vi "Autonomous Independent.vi"() -> ()   [LabVIEW 2014]
doc: "This VI is called when autonomous begins, and will automatically be terminated when autonomous ends. You can carry out timed or sensor driven robot movement independently without needing to return to the caller."
uses:
  <vilib>/Rock Robotics/WPI/Joystick/WPI_JoystickGetSetRefNum.vi
  <vilib>/Rock Robotics/Network Tables/SD Read Boolean.vi
panel:
  in  "input cluster":T1
  # "Be sure to right-click and choose Data Operations>>Make Current Value default if you want to save the array values with the VI"
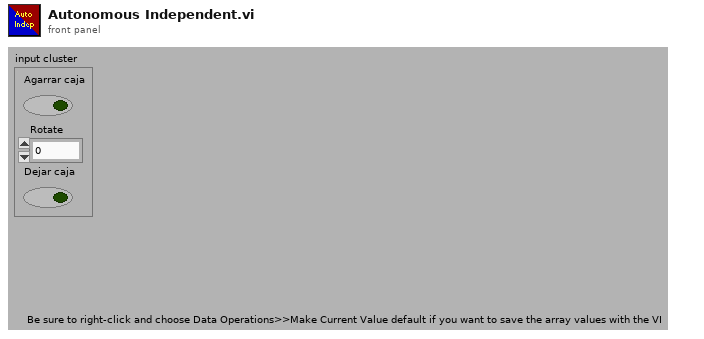
[diagram p1: front panel]
types:
  T1 = cluster{"Agarrar caja":bool, "Rotate":dbl, "Dejar caja":bool}
  T2 = enum16{"GTFO", "Drop the beat", "Moonwalk", "Stare at the box", "Kiss the Wall", "Take that motherfucker"}
  T3 = typedef "WPI_JoystickDevRef.ctl" = cluster{"Device":T4}
  T4 = typedef "WPI_JoystickDeviceEnum.ctl" = enum16{"USB 0", "USB 1", "USB 2", "USB 3", "USB 4", "USB 5"}
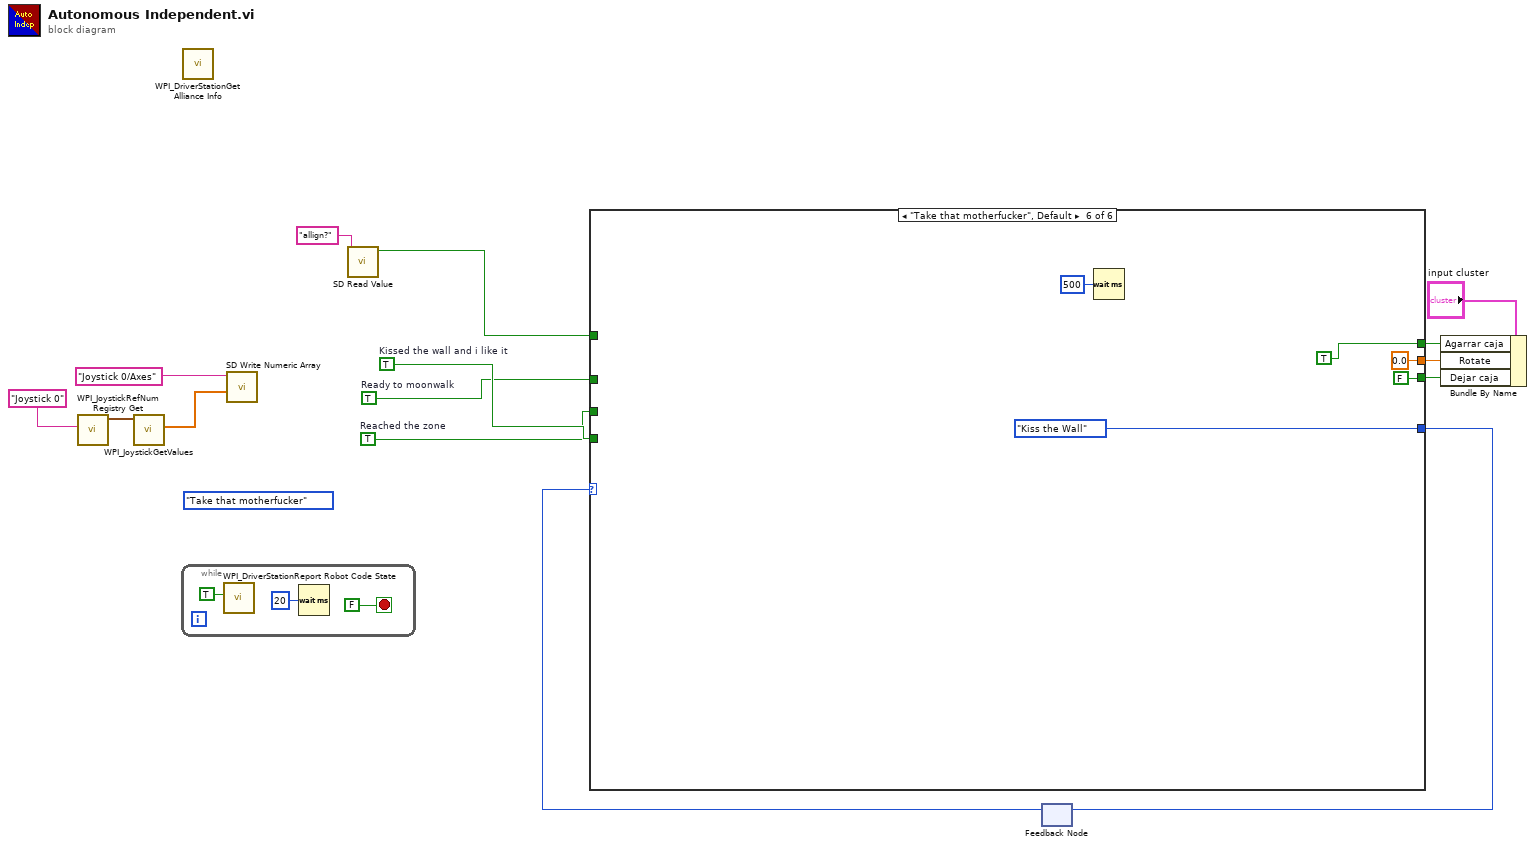
[diagram p0: block diagram]
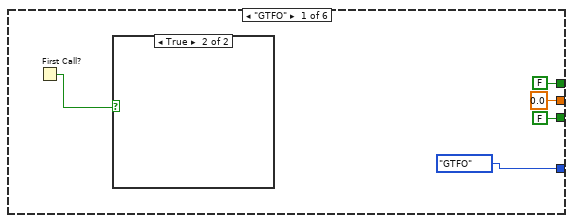
[diagram p2: hidden frame]
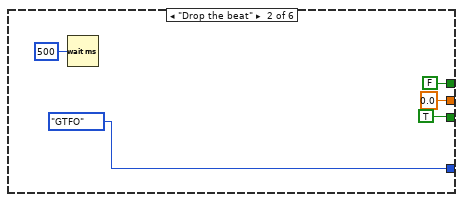
[diagram p4: hidden frame]
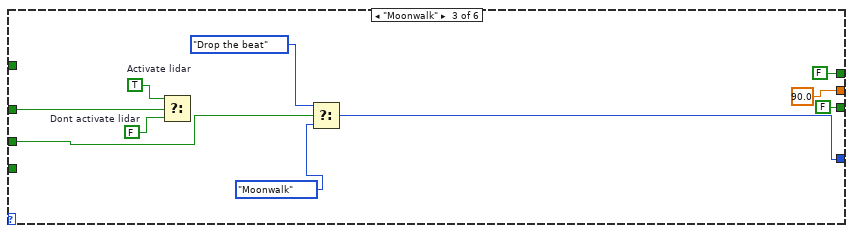
[diagram p5: hidden frame]
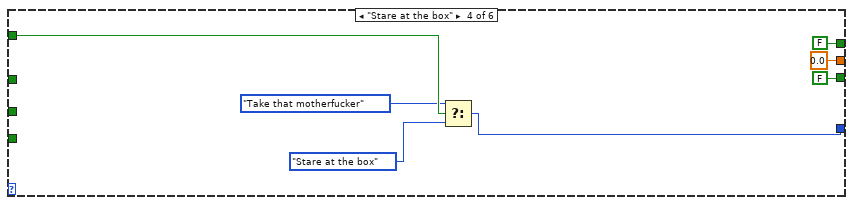
[diagram p6: hidden frame]
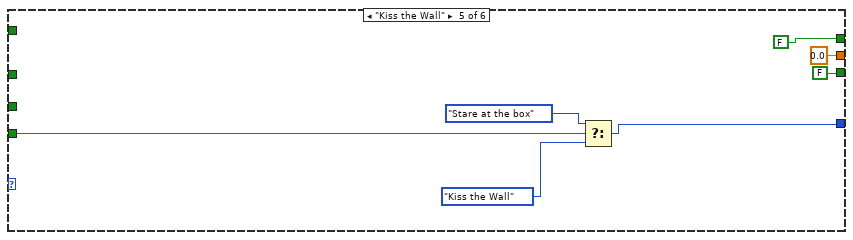
[diagram p7: hidden frame]
diagram:
  w2 = TRUE  # Reached the zone
  w3 = TRUE  # Ready to moonwalk
  w7 = TRUE  # Kissed the wall and i like it
  (unwired) T2."Take that motherfucker"
  n1 = call <vilib>:"WPI_JoystickRefNum Registry Get.vi"("refnum name"="Joystick 0") -> ("JoystickDevRef"=w14:T3)  [unwired: 1 in, 9 out]
  n2 = call <vilib>:"WPI_JoystickGetValues.vi"("JoystickDevRef"=w14) -> ("Axes"=w12:dbl[])  [unwired: 6 in, 4 out]
  n3 = while {
    stop <- FALSE stop-if-true
    n4 = call <vilib>:"WPI_DriverStationReport Robot Code State.vi"("Autonomous"=TRUE) -> ()  [unwired: 10 in, 1 out]
    n5 = Wait (ms)(milliseconds to wait=u32 20) -> ()  [unwired: 1 out]
  }
  n6 = call <vilib>:"WPI_DriverStationGet Alliance Info.vi"() -> ()  [unwired: 12 out]
  n7 = call <vilib>:"SD Write Numeric Array.vi"("Numeric Array"=w12, "Name"="Joystick 0/Axes") -> ()  [unwired: 8 in, 2 out]
  n8 = call-poly <vilib>:"SD Read Value.vi"("Name"="allign?") -> ("Boolean"=w5:bool)  [unwired: 8 in, 2 out]
  n9 = feedback #1() -> (w8:T2)  [unwired: 1 in]
  n10 = case shown="\"Take that motherfucker\", Default" w8 {
    tunnel: [FALSE FALSE FALSE FALSE FALSE TRUE] -> w10
    tunnel: [T2."GTFO" T2."GTFO" w31 w42 w50 T2."Kiss the Wall"] -> w9
    tunnel: w7 -> [_ _ _ _ w48 _]
    tunnel: w5 -> [_ _ _ w45 _ _]
    tunnel: [0.0 0.0 90.0 0.0 0.0 0.0] -> w4
    tunnel: w3 -> [_ _ w37 _ _ _]
    tunnel: w2 -> [_ _ w34 _ _ _]
    tunnel: [FALSE TRUE FALSE FALSE FALSE FALSE] -> w1
    frame "GTFO" {
      n11 = First Call?() -> (First Call?: T/F=w19:bool)
      n12 = case shown="True" w19 {
        frame False {
        }
        frame True {
        }
      }
    }
    frame "Drop the beat" {
      n13 = Wait (ms)(milliseconds to wait=u32 500) -> ()  [unwired: 1 out]
    }
    frame "Moonwalk" {
      w35 = TRUE  # Activate lidar
      w36 = FALSE  # Dont activate lidar
      n14 = Select(t=w35, s=w37, f=w36) -> ()  [unwired: 1 out]
      n15 = Select(t=T2."Drop the beat", s=w34, f=T2."Moonwalk") -> (s? t:f=w31:T2)
    }
    frame "Stare at the box" {
      n16 = Select(t=T2."Take that motherfucker", s=w45, f=T2."Stare at the box") -> (s? t:f=w42:T2)
    }
    frame "Kiss the Wall" {
      n17 = Select(t=T2."Stare at the box", s=w48, f=T2."Kiss the Wall") -> (s? t:f=w50:T2)
    }
    frame "Take that motherfucker", Default {
      n18 = Wait (ms)(milliseconds to wait=u32 500) -> ()  [unwired: 1 out]
    }
  }
  n19 = feedback-in #1(w9) -> ()
  n20 = Bundle By Name(cluster="input cluster", "Agarrar caja"=w10, "Rotate"=w4, "Dejar caja"=w1) -> ()  [unwired: 1 out]
